vi "enqueueTelToComponent.vi"(8 "error in (no error)":errorcluster, 10 "Elements to enqueue":string, 11 "TcpServerTel in":refnum<class "TcpServerTel.lvclass">) -> (0 "error out":errorcluster, 1 "timeoutQueueTcpClientFromDds":bool, 2 "overflowQueueTcpClientFromDds":bool, 3 "TcpServerTel out":refnum<class "TcpServerTel.lvclass">)   [LabVIEW 2018, in "TcpServerTel.lvclass"]
doc: "Enqueue elements into the queueTcpClientFromDds through Lossy Enqueue Element function or Enqueue Element function. This selection is done in the configServer.vi. This telemetry comes from TCP Client and is sent to LabVIEW Component."
uses:
  TcpServerTel.lvclass
  home/pcortes/github/ts_labview_tcp_json/src/TcpServerBase/TcpServerBase.lvclass
  TcpServerTel.lvclass/TcpServerTel.ctl
  TcpServerBase/TcpServerBase.lvclass
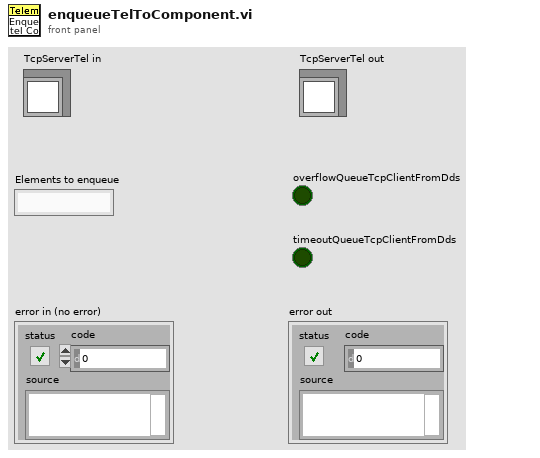
[diagram p1: front panel]
types:
  T1 = typedef "TcpServerTel.lvclass/enqueueOptionsTypeDef.ctl" = enum16{"lossy enqueue", "normal enqueue"}
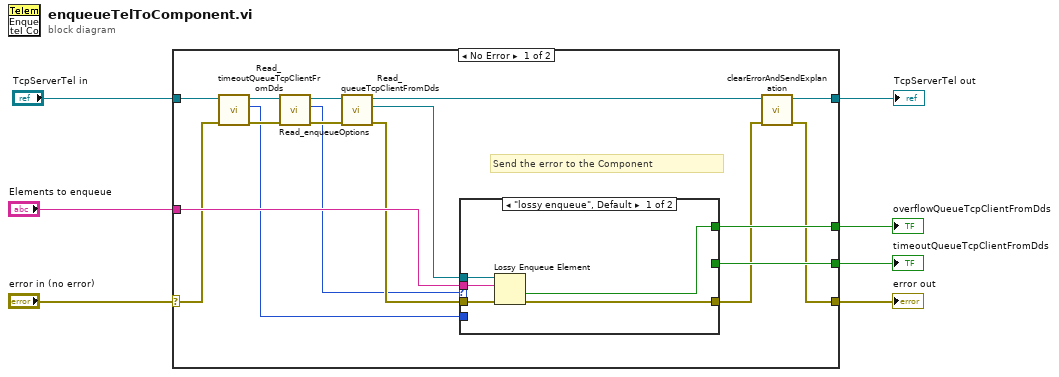
[diagram p0: block diagram]
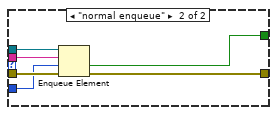
[diagram p2: hidden frame]
diagram:
  n1 = case shown="No Error" "error in (no error)" {
    selector: "error in (no error)" -> [w17 w36]
    tunnel: [w8 w36] -> w7
    tunnel: "Elements to enqueue" -> [w24 _]
    tunnel: [w23 _] -> w5
    tunnel: "TcpServerTel in" -> [w14 w37]
    tunnel: [w10 w37] -> w3
    tunnel: [w11 _] -> w1
    frame No Error {
      # "Send the error to the Component"
      n2 = call "Read_timeoutQueueTcpClientFromDds.vi"("error in (no error)"=w17, "TcpServerTel in"=w14) -> ("error out"=w15:errorcluster, "timeoutQueueTcpClientFromDds"=w12:i32, "TcpServerTel out"=w13:refnum<class "TcpServerTel.lvclass">)  [unwired: 7 in]
      n3 = call "Read_enqueueOptions.vi"("error in (no error)"=w15, "TcpServerTel in"=w13) -> ("error out"=w18:errorcluster, "EnqueueOptions"=w16:T1, "TcpServerTel out"=w19:refnum<class "TcpServerTel.lvclass">)  [unwired: 7 in]
      n4 = call "Read_queueTcpClientFromDds.vi"("error in (no error)"=w18, "TcpServerTel in"=w19) -> ("error out"=w20:errorcluster, "queueTcpClientFromDds"=w22:refnum<queue>, "TcpServerTel out"=w21:refnum<class "TcpServerTel.lvclass">)  [unwired: 7 in]
      n5 = case shown="\"lossy enqueue\", Default" w16 {
        tunnel: [w29 w34] -> w9
        tunnel: w20 -> [w28 w35]
        tunnel: w24 -> [w27 w32]
        tunnel: w22 -> [w26 w33]
        tunnel: [w25 _] -> w23
        tunnel: w12 -> [_ w31]
        tunnel: [_ w30] -> w11
        frame "lossy enqueue", Default {
          n6 = Lossy Enqueue Element(queue=w26, element=w27, error in (no error)=w28) -> (overflow?=w25:bool, error out=w29:errorcluster)  [unwired: 2 out]
        }
        frame "normal enqueue" {
          n7 = Enqueue Element(queue=w33, element=w32, timeout in ms (-1)=w31, error in (no error)=w35) -> (timed out?=w30:bool, error out=w34:errorcluster)  [unwired: 1 out]
        }
      }
      n8 = call "clearErrorAndSendExplanation.vi"("error in (no error)"=w9, "TcpServerBase in"=w21) -> ("error out"=w8:errorcluster, "TcpServerBase out"=w10:refnum<class "TcpServerTel.lvclass">)  [unwired: 8 in]
    }
    frame Error {
    }
  }
  "error out" <- w7
  "overflowQueueTcpClientFromDds" <- w5
  "TcpServerTel out" <- w3
  "timeoutQueueTcpClientFromDds" <- w1
